vi "BUILD_read vip token.vi"(10 "regular expression":string, 11 "data":string) -> (3 "trimmed string":string)   [LabVIEW 2010]
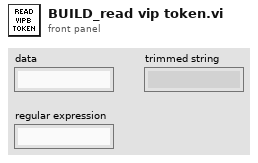
[diagram p1: front panel]
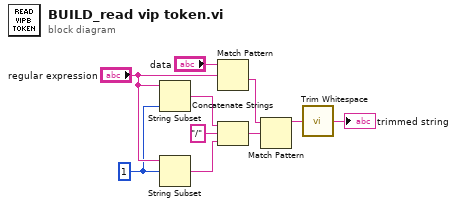
[diagram p0: block diagram]
diagram:
  w1 = 1 ("length (rest)")
  n1 = String Subset(string="regular expression", length (rest)=w1) -> (substring=w2:string)  [unwired: 1 in]
  n2 = String Subset(string="regular expression", offset (0)=w1) -> (substring=w3:string)  [unwired: 1 in]
  n3 = Match Pattern(string="data", regular expression="regular expression") -> (after substring=w9:string)  [unwired: 1 in, 3 out]
  n4 = Concatenate Strings(w2, "/" ("string"), w3) -> (w5:string)
  n5 = Match Pattern(string=w9, regular expression=w5) -> (before substring=w6:string)  [unwired: 1 in, 3 out]
  n6 = call <vilib>:"Trim Whitespace.vi"("string"=w6) -> ("trimmed string"=→"trimmed string":string)  [unwired: 1 in]
